vi "json Create.vi"(8 "error in (no error)":errorcluster, 10 "JSON String":string) -> (0 "error out":errorcluster, 3 "JSON Document out":refnum<class "JSON Document.lvclass">)   [LabVIEW 2015, in "JSON Document.lvclass"]
uses:
  JSON Document.lvclass
  JSON Document.lvclass/JSON Document.ctl
  rapidjson wrapper/rapidjson wrapper.lvlib
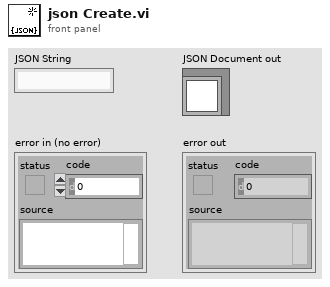
[diagram p1: front panel]
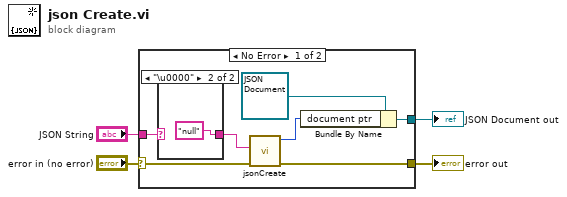
[diagram p0: block diagram]
diagram:
  n1 = case shown="No Error" "error in (no error)" {
    selector: "error in (no error)" -> [w11 w14]
    tunnel: [w10 w14] -> w3
    tunnel: "JSON String" -> [w6 _]
    tunnel: [w7 _] -> w1
    frame No Error {
      n2 = case shown="\"\"" w6 {
        selector: w6 -> [w12 _]
        tunnel: [w12 "null" ("JSON String")] -> w5
        frame Default {
        }
        frame "\u0000" {
        }
      }
      n3 = call "jsonCreate.vi"("error in (no error)"=w11, "json"=w5) -> ("error out"=w10:errorcluster, "d"=w8:i64)  [unwired: 8 in]
      n4 = Bundle By Name(cluster=refnum<class "JSON Document.lvclass"> refnum ("JSON Document.lvclass"), "document ptr"=w8) -> (w7:refnum<class "JSON Document.lvclass">)
    }
    frame Error {
    }
  }
  "error out" <- w3
  "JSON Document out" <- w1
